vi "Inspect Test Pattern.vi"() -> ()   [LabVIEW 2016]
panel:
  in  "offset (0)":i64=124993
  out "Waveform Graph":waveform(dbl)[](graph)
  in  "Interpolation":dbl=64.0
  in  "channel name":string[](array[string])=["I", "Vavg", "Case"]
  in  "File Path Control":path=path "C:/Data/September_2017/092917/p006_092917.tdms"
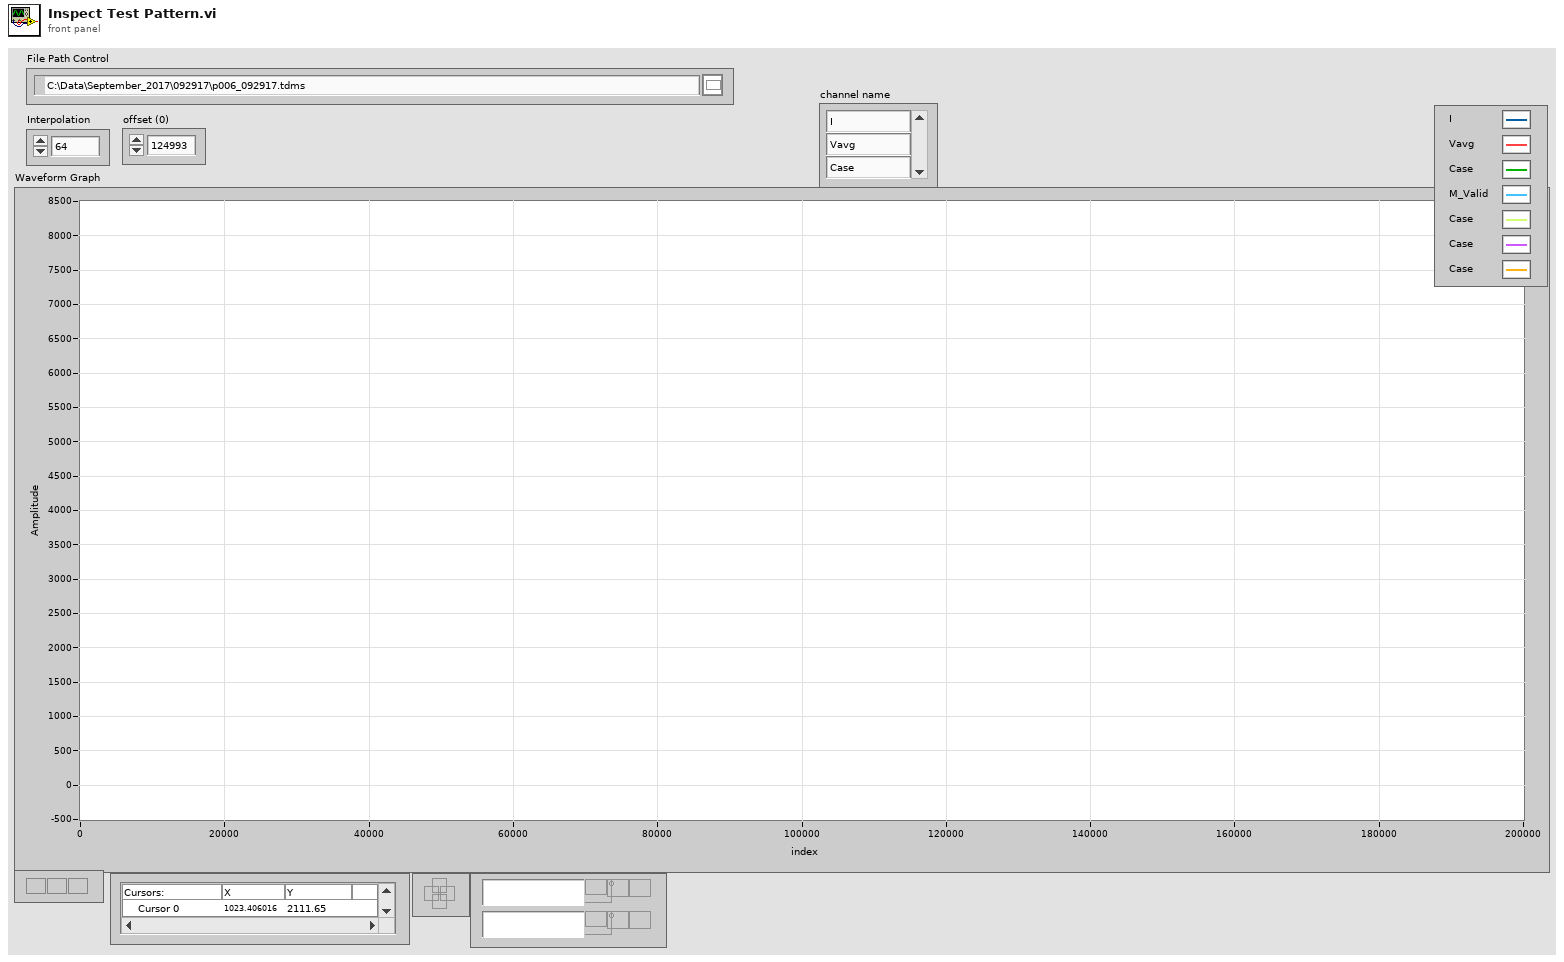
[diagram p1: front panel]
types:
  T1 = enum16{"open", "open or create", "create or replace", "create", "open (read-only)"}
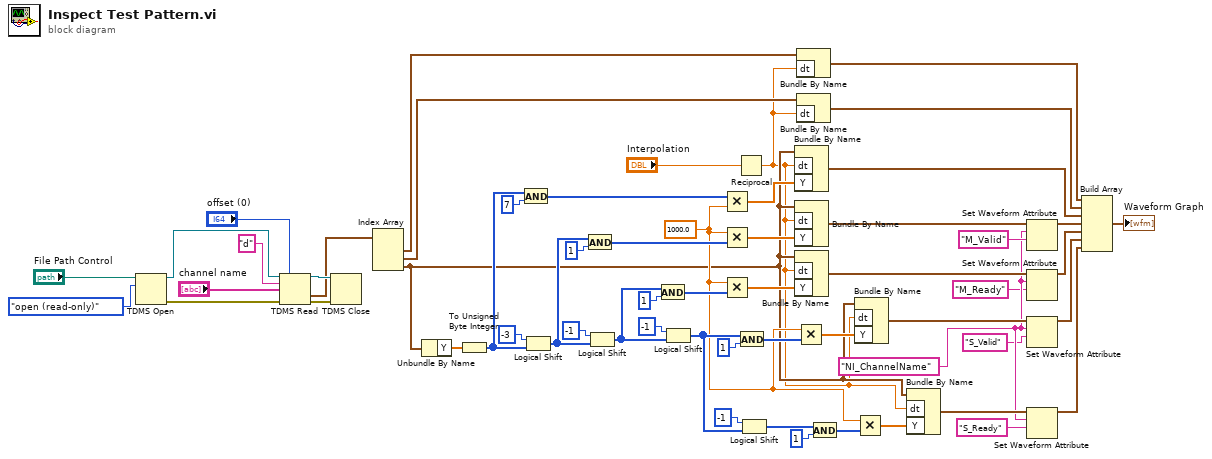
[diagram p0: block diagram]
diagram:
  w4 = "NI_ChannelName" ("name")
  w14 = 1000.0
  n1 = TDMS Open(10:T1."open (read-only)" ("operation (0:open)"), 11:"File Path Control") -> (0:w56:errorcluster, 3:w57:refnum<k34>)  [unwired: 5 in]
  n2 = TDMS Read(0:w57, 1:"offset (0)", 5:"d" ("group name"), 7:"channel name", 11:w56) -> (4:w52:refnum<k34>, 10:w45:waveform(dbl)[], 15:w53:errorcluster)  [unwired: 3 in, 3 out]
  n3 = TDMS Close(8:w53, 11:w52) -> ()  [unwired: 2 out]
  n4 = Index Array(array=w45) -> (element #1=w42:waveform(dbl), element #2=w46:waveform(dbl), element #3=w13:waveform(dbl))  [unwired: 3 in]
  n5 = Unbundle By Name(w13) -> ("Y"=w41:dbl[])
  n6 = To Unsigned Byte Integer(number=w41) -> (unsigned 8bit integer=w37:u8[])
  n7 = And(x=w37, y=7) -> (x .and. y?=w39:i32[])
  n8 = Logical Shift(y=-3, x=w37) -> (x << y=w28:u8[])
  n9 = And(x=w28, y=1) -> (x .and. y?=w35:i32[])
  n10 = Logical Shift(y=-1, x=w28) -> (x << y=w16:u8[])
  n11 = And(x=w16, y=1) -> (x .and. y?=w30:i32[])
  n12 = Logical Shift(y=-1, x=w16) -> (x << y=w15:u8[])
  n13 = Multiply(x=w39, y=w14) -> (x*y=w38:dbl[])
  n14 = Multiply(x=w14, y=w35) -> (x*y=w33:dbl[])
  n15 = Multiply(x=w14, y=w30) -> (x*y=w27:dbl[])
  n16 = Reciprocal(x="Interpolation") -> (1/x=w12:dbl)
  n17 = And(x=w15, y=1) -> (x .and. y?=w23:i32[])
  n18 = Logical Shift(y=-1, x=w15) -> (x << y=w20:u8[])
  n19 = Bundle By Name(cluster=w13, "dt"=w12, "Y"=w38) -> (w49:waveform(dbl))
  n20 = Bundle By Name(cluster=w13, "dt"=w12, "Y"=w33) -> (w32:waveform(dbl))
  n21 = Bundle By Name(cluster=w13, "dt"=w12, "Y"=w27) -> (w26:waveform(dbl))
  n22 = Multiply(x=w14, y=w23) -> (x*y=w25:dbl[])
  n23 = Bundle By Name(cluster=w42, "dt"=w12) -> (w43:waveform(dbl))
  n24 = Bundle By Name(cluster=w46, "dt"=w12) -> (w44:waveform(dbl))
  n25 = And(x=w20, y=1) -> (x .and. y?=w19:i32[])
  n26 = Bundle By Name(cluster=w13, "dt"=w12, "Y"=w25) -> (w11:waveform(dbl))
  n27 = Multiply(x=w14, y=w19) -> (x*y=w17:dbl[])
  n28 = Bundle By Name(cluster=w13, "dt"=w12, "Y"=w17) -> (w10:waveform(dbl))
  n29 = Set Waveform Attribute(5:"M_Valid" ("name"), 6:w4, 7:w32) -> (3:w9:waveform(dbl))  [unwired: 1 in, 2 out]
  n30 = Set Waveform Attribute(5:"M_Ready" ("name"), 6:w4, 7:w26) -> (3:w8:waveform(dbl))  [unwired: 1 in, 2 out]
  n31 = Set Waveform Attribute(5:"S_Valid" ("name"), 6:w4, 7:w11) -> (3:w7:waveform(dbl))  [unwired: 1 in, 2 out]
  n32 = Set Waveform Attribute(5:"S_Ready" ("name"), 6:w4, 7:w10) -> (3:w6:waveform(dbl))  [unwired: 1 in, 2 out]
  n33 = Build Array(w43, w44, w49, w9, w8, w7, w6) -> (→"Waveform Graph":waveform(dbl)[])
